vi "Set Active Item.vi"(9 "Display Items":T1[](array[typedef]), 10 "NewVal":string[](array[string]), 11 "TreeControl in":refnum<vi>) -> (3 "TreeControl out":refnum<vi>)   [LabVIEW 2023]
doc: "The active item in a tree is the basis for arrow key navigation, so it must be set when the value is change/ However, we get an error when a value is unset, as we can't set the tag to a value that isn't displayed, or a blank. Take care of all the details here.\n\nIf there is no current selection, the active item is set to the first displayed item."
uses:
  cluster/Cluster Element Description.ctl
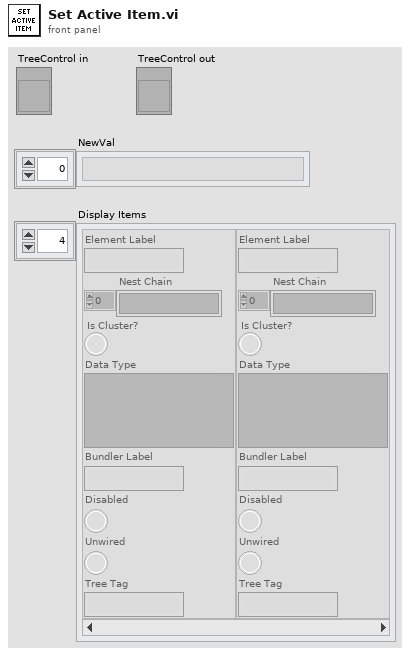
[diagram p1: front panel]
types:
  T1 = typedef "Cluster Element Description.ctl" = cluster{"Element Label":string, "Nest Chain":string[], "Is Cluster?":bool, "Data Type":variant, "Bundler Label":string, "Disabled":bool, "Unwired":bool, "Tree Tag":string}
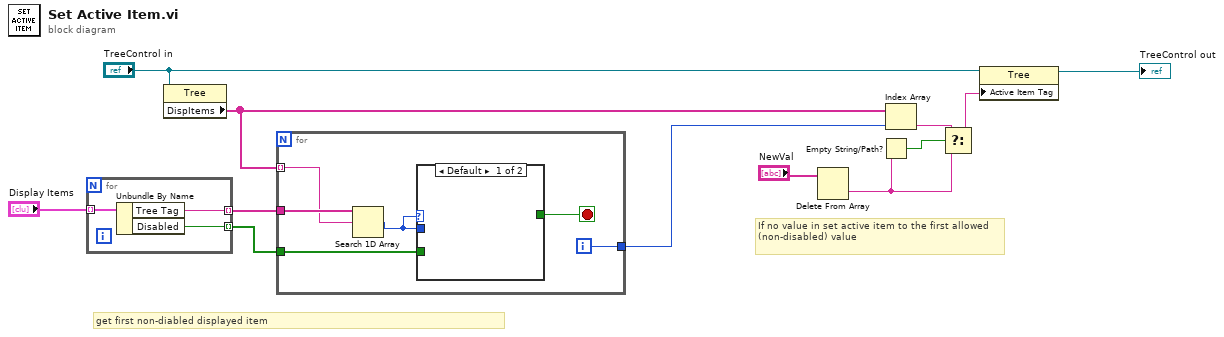
[diagram p0: block diagram]
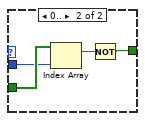
[diagram p2: hidden frame]
diagram:
  # "get first non-diabled displayed item"
  # "If no value in set active item to the first allowed (non-disabled) value"
  n1 = for {
    tunnel: "Display Items" -> [w15] mode=indexing
    tunnel: [w14] -> w3 mode=indexing
    tunnel: [w13] -> w2 mode=indexing
    n2 = Unbundle By Name(w15) -> ("Tree Tag"=w14:string, "Disabled"=w13:bool)
  }
  n3 = property class="Tree"(reference="TreeControl in") -> ("DispItems"=w5:string[])  [unwired: 1 in, 2 out]
  n4 = for {
    tunnel: w5 -> [w20] mode=indexing
    tunnel: w3 -> [w21]
    tunnel: w2 -> [w19]
    tunnel: [w16] -> w1
    i -> [w16]
    stop <- w17 stop-if-true
    n5 = Search 1D Array(1D array=w21, element=w20) -> (index of element=w18:i32)  [unwired: 1 in]
    n6 = case shown="Default" w18 {
      tunnel: w19 -> [_ w25]
      tunnel: w18 -> [_ w24]
      tunnel: [_ w22] -> w17
      frame Default {
      }
      frame 0.. {
        n7 = Index Array(array=w25, index=w24) -> (element=w23:bool)
        n8 = Not(x=w23) -> (.not. x?=w22:bool)
      }
    }
  }
  n9 = Delete From Array(array="NewVal") -> (deleted portion=w8:string)  [unwired: 2 in, 1 out]
  n10 = Empty String/Path?(string/path=w8) -> (empty?=w7:bool)
  n11 = Index Array(array=w5, index=w1) -> (element=w9:string)
  n12 = Select(t=w9, s=w7, f=w8) -> (s? t:f=w6:string)
  n13 = property class="Tree"(reference="TreeControl in", "Active Item Tag"=w6) -> (reference out=→"TreeControl out":refnum<vi>)  [unwired: 1 in, 1 out]
